vi "ABOUT STRING.vi"() -> ()   [LabVIEW 2025]
uses:
  <vilib>/Utility/error.llb/whitespace.ctl
  <vilib>/Utility/error.llb/Trim Whitespace One-Sided.vi
  <vilib>/regexp/Match Regular Expression.xnode
panel:
  out "error out":errorcluster
  out "offset past match 2":i32
  out "after match":string
  out "whole match":string
  out "before match":string
  in  "multiline? (F)":bool
  in  "ignore case? (F)":bool
  in  "error in":errorcluster
  in  "offset (0)":i32
  in  "regular expression 2":string
  in  "input string 2":string
  out "offset past match":i32
  out "after substring":string
  out "match substring":string
  out "before substring":string
  in  "regular expression":string
  in  "string":string
  out "offset past replacement":i32
  out "number of replacements":i32
  out "result string":string
  in  "input string":string
  out "replaced substring":string
  out "result":string
  in  "replace character":string
  in  "A":string
  out "b":string
  in  "A":string
  out "trimmed string":string
  in  "A":string
  out "substring":string
  in  "A":string
  out "merge string":string
  in  "A 2":string
  in  "A":string
  out "length of the string":i32
  in  "A":string
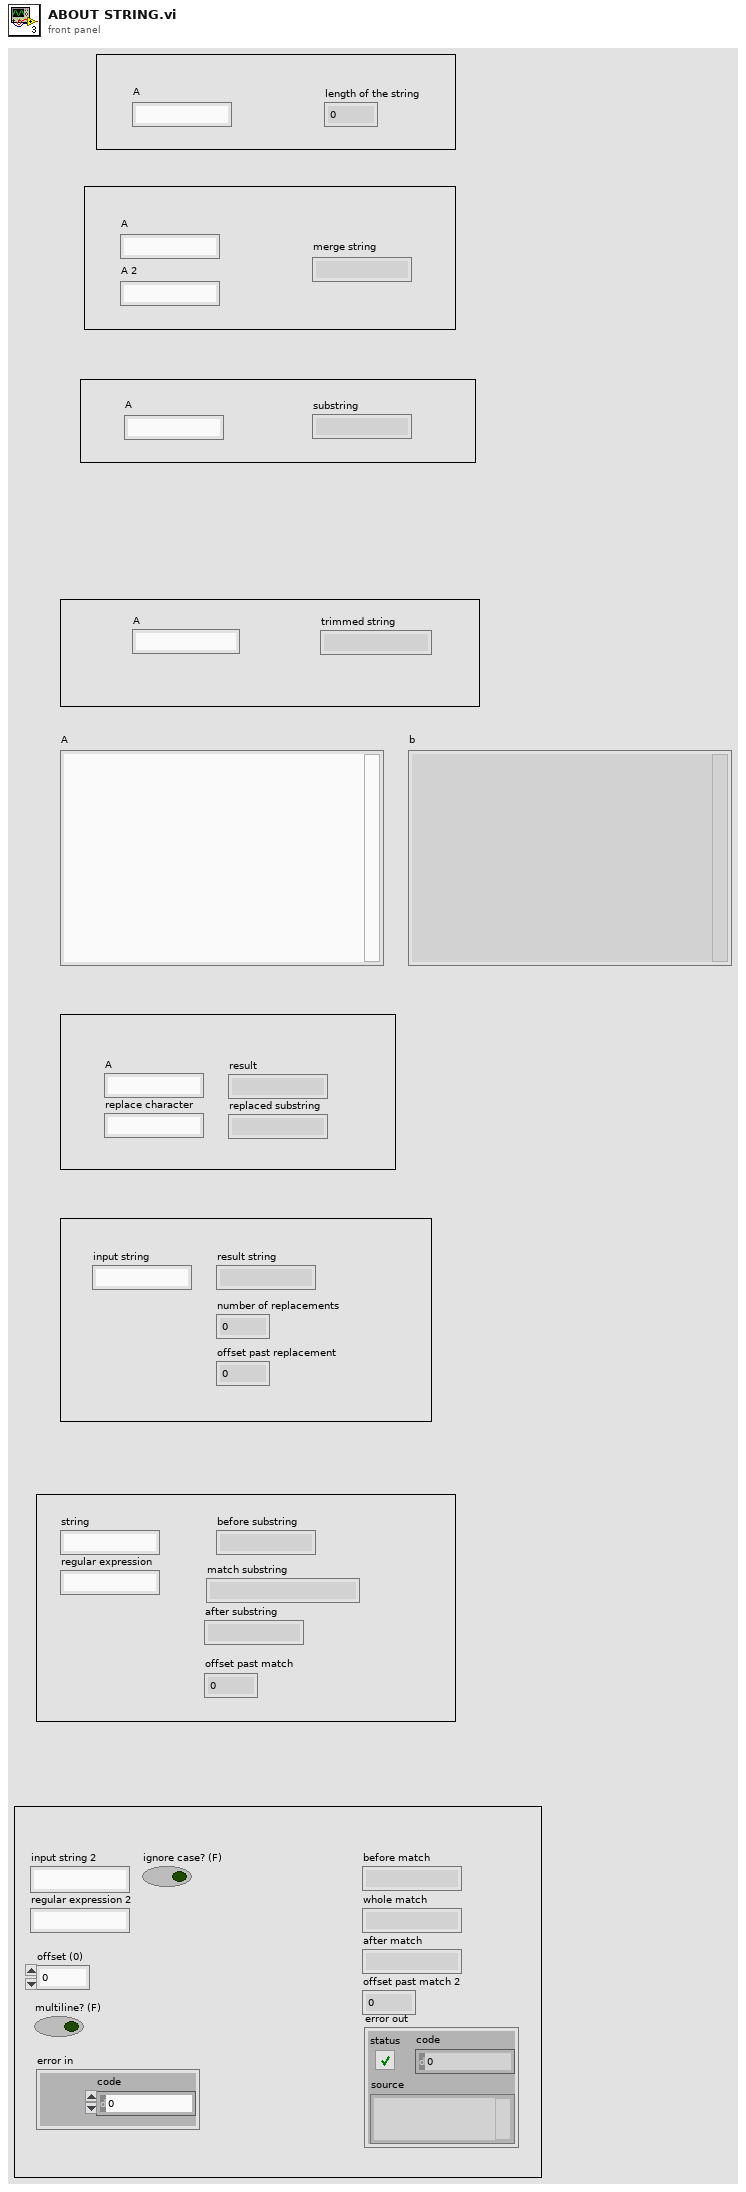
[diagram p1: front panel]
types:
  T1 = enum16{"Native", "Native Command Line", "UNIX", "Macintosh", "DOS"}
  T2 = typedef "whitespace.ctl" = u16
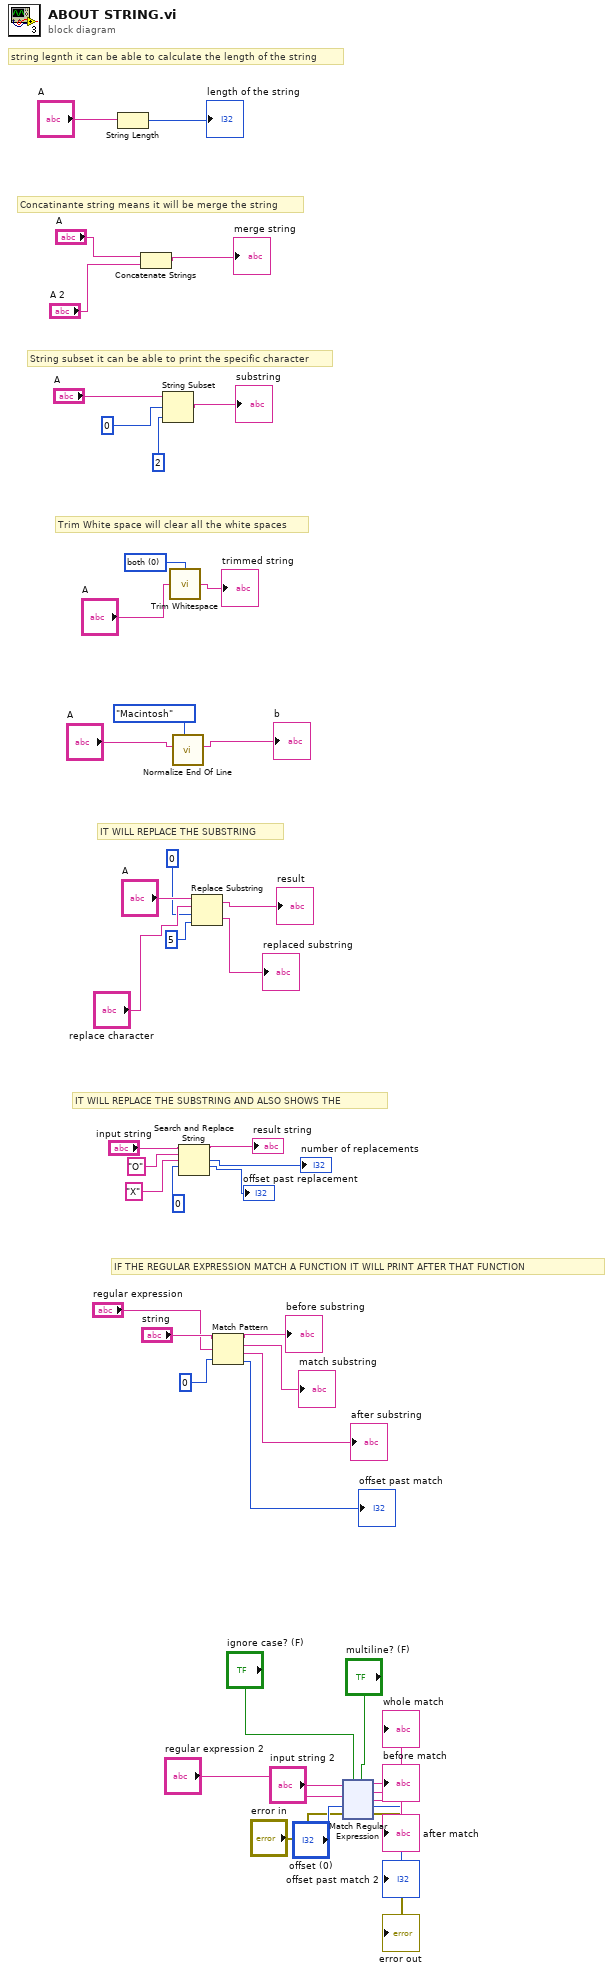
[diagram p0: block diagram]
diagram:
  w37 = T2 0 items=["both", "start of string", "end of string"] ("location (both)")
  # "IF THE REGULAR EXPRESSION MATCH A FUNCTION IT WILL PRINT AFTER THAT FUNCTION"
  # "IT WILL REPLACE THE SUBSTRING AND ALSO SHOWS THE"
  # "IT WILL REPLACE THE SUBSTRING"
  # "Trim White space will clear all the white spaces"
  # "String subset it can be able to print the specific character"
  # "Concatinante string means it will be merge the string"
  # "string legnth it can be able to calculate the length of the string"
  n1 = String Length(string="A") -> (length=→"length of the string":i32)
  n2 = Concatenate Strings("A", "A 2") -> (→"merge string":string)
  n3 = String Subset(string="A", offset (0)=0, length (rest)=2 ("length (rest)")) -> (substring=→"substring":string)
  n4 = call <vilib>:"Trim Whitespace.vi"("string"="A", "location (both)"=w37) -> ("trimmed string"=→"trimmed string":string)
  n5 = call <vilib>:"Normalize End Of Line.vi"("end of line (Native)"=T1."Macintosh", "string in"="A") -> ("string out"=→"b":string)  [unwired: 6 in]
  n6 = Search and Replace String(input string="input string", search string="O", replace string="X" ("replace string (\"\")"), offset=0 ("offset (0)")) -> (result string=→"result string":string, number of replacements=→"number of replacements":i32, offset past replacement=→"offset past replacement":i32)  [unwired: 4 in, 1 out]
  n7 = Replace Substring(2:5 ("length (len. of substring)"), 3:0 ("offset (0)"), 4:"replace character", 5:"A") -> (0:→"replaced substring":string, 1:→"result":string)
  n8 = Match Pattern(string="string", regular expression="regular expression", offset (0)=0) -> (before substring=→"before substring":string, match substring=→"match substring":string, after substring=→"after substring":string, offset past match=→"offset past match":i32)
  n9 = xnode "Match Regular Expression"("input string"="input string 2", "regular expression"="regular expression 2", "offset (0)"="offset (0)", "error in"="error in", "ignore case? (F)"="ignore case? (F)", "multiline? (F)"="multiline? (F)") -> ("before match"=→"before match":string, "whole match"=→"whole match":string, "after match"=→"after match":string, "offset past match"=→"offset past match 2":i32, "error out"=→"error out":errorcluster)
